vi "Test_PT1_discrete.vi"() -> ()   [LabVIEW 2022 SP3]
uses:
  <vilib>/gmath/NI_Gmath.lvlib
panel:
  in  "Tcyc":dbl=9284646.0 format="%#_13g"
  in  "Gain":dbl format="%#_13g"
  out "Waveform Graph":dbl[][](graph)
  in  "Operation":enum16{"Lag", "rapid adjustment"}(ring)
  in  "T":dbl format="%#_13g"
  in  "stop":bool
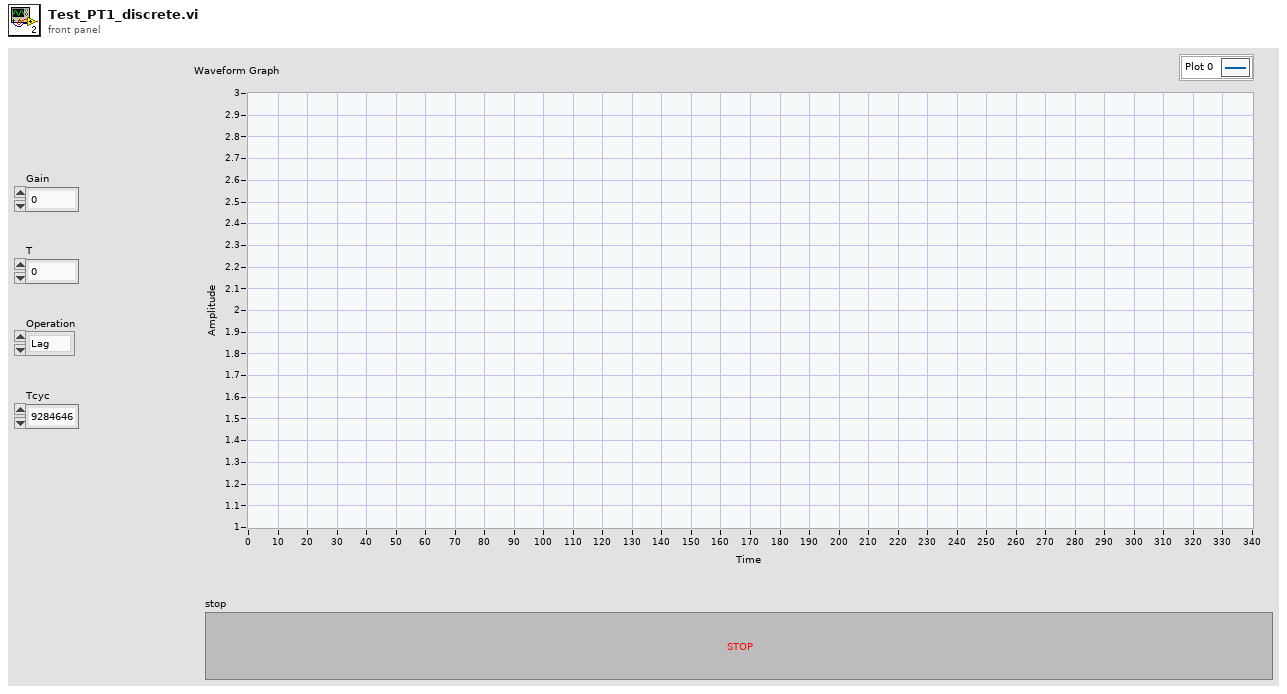
[diagram p1: front panel]
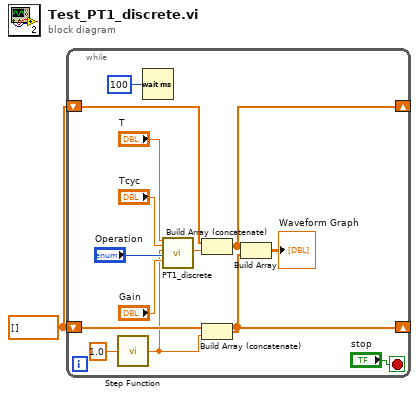
[diagram p0: block diagram]
diagram:
  w1 = dbl[] []
  n1 = while {
    shift-right: [w8] -> _
    shift-left: w1 -> [w10]
    shift-right: [w7] -> _
    shift-left: w1 -> [w9]
    stop <- "stop" stop-if-true
    n2 = call <vilib>:"Step Function.vi"("x"=1.0) -> ("step(x)"=w2:dbl)
    n3 = Wait (ms)(milliseconds to wait=u32 100) -> ()  [unwired: 1 out]
    n4 = call "PT1_discrete.vi"("T"="T", "Tcyc"="Tcyc", "AI1"=w2, "Operation"="Operation", "Gain"="Gain") -> ("AO1"=w11:dbl)  [unwired: 13 in, 1 out]
    n5 = Build Array (concatenate)(w10, w11) -> (w8:dbl[])
    n6 = Build Array (concatenate)(w9, w2) -> (w7:dbl[])
    n7 = Build Array(w8, w7) -> (→"Waveform Graph":dbl[][])
  }
